vi "LatManClicks.vi"(9 "nMilliseconds":i32=2000, 10 "error in (no error)":errorcluster, 11 "On/OFF":bool) -> (2 "error out":errorcluster)   [LabVIEW 2014]
panel:
  in  "AutoItX3Lib.IAutoItX3":refnum<k7>
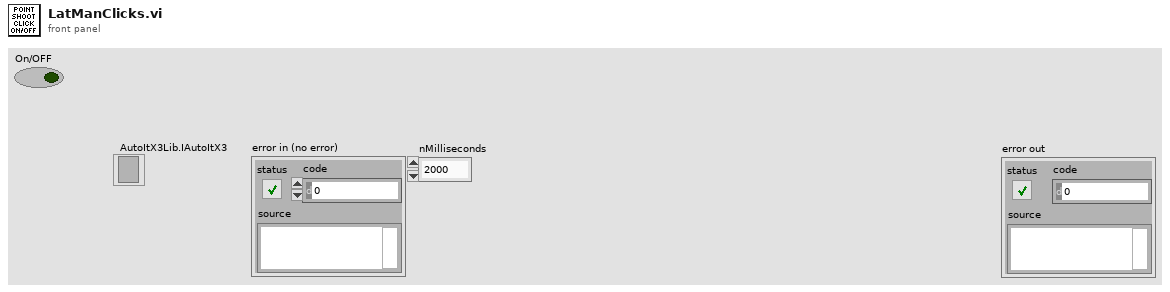
[diagram p1: front panel]
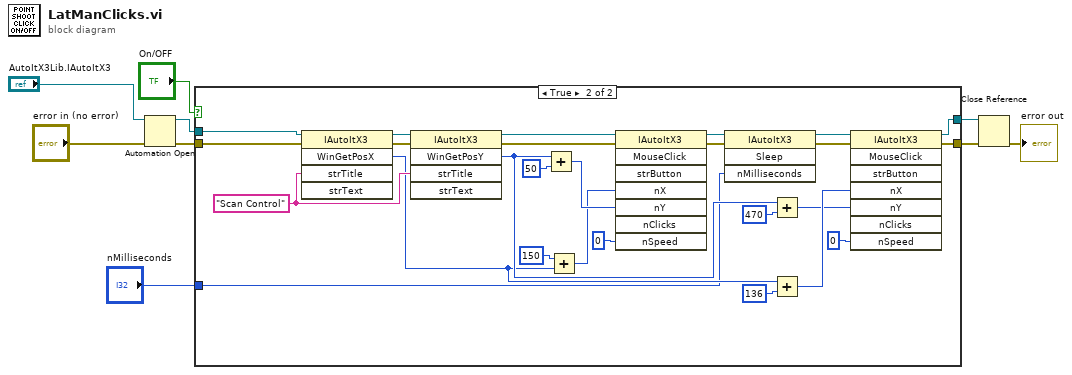
[diagram p0: block diagram]
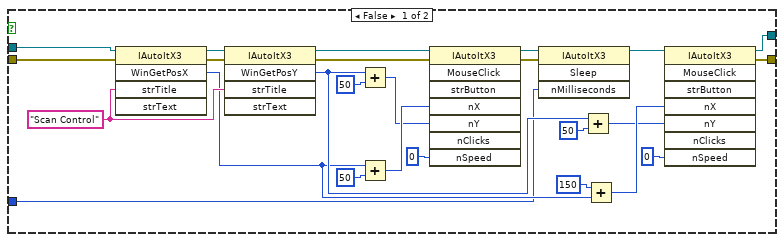
[diagram p2: hidden frame]
diagram:
  n1 = Automation Open(error in (no error)="error in (no error)", Automation Refnum="AutoItX3Lib.IAutoItX3") -> (Automation Refnum=w7:refnum<k7>, error out=w6:errorcluster)  [unwired: 2 in]
  n2 = case shown="True" "On/OFF" {
    tunnel: w7 -> [w32 w60]
    tunnel: w6 -> [w31 w59]
    tunnel: [w25 w50] -> w5
    tunnel: [w13 w49] -> w4
    tunnel: "nMilliseconds" -> [w10 w35]
    frame False {
      w24 = "Scan Control" ("strTitle")
      n3 = invoke class="IAutoItX3" method="WinGetPosX"(reference=w32, error in=w31, "strTitle"=w24) -> (reference out=w30:refnum<k7>, error out=w27:errorcluster, "WinGetPosX"=w22:i32)  [unwired: 2 in, 2 out]
      n4 = invoke class="IAutoItX3" method="WinGetPosY"(reference=w30, error in=w27, "strTitle"=w24) -> (reference out=w29:refnum<k7>, error out=w28:errorcluster, "WinGetPosY"=w23:i32)  [unwired: 2 in, 2 out]
      n5 = Add(x=w23, y=50) -> (x+y=w18:i32)
      n6 = Add(x=w22, y=50) -> (x+y=w19:i32)
      n7 = invoke class="IAutoItX3" method="MouseClick"(reference=w29, error in=w28, "nX"=w19, "nY"=w18, "nSpeed"=0) -> (reference out=w34:refnum<k7>, error out=w33:errorcluster)  [unwired: 3 in, 6 out]
      n8 = invoke class="IAutoItX3" method="Sleep"(reference=w34, error in=w33, "nMilliseconds"=w10) -> (reference out=w26:refnum<k7>)  [unwired: 1 in, 3 out]
      n9 = Add(x=w23, y=50) -> (x+y=w20:i32)
      n10 = Add(x=150, y=w22) -> (x+y=w21:i32)
      n11 = invoke class="IAutoItX3" method="MouseClick"(reference=w26, "nX"=w21, "nY"=w20, "nSpeed"=0) -> (reference out=w25:refnum<k7>, error out=w13:errorcluster)  [unwired: 4 in, 6 out]
    }
    frame True {
      w56 = "Scan Control" ("strTitle")
      n12 = invoke class="IAutoItX3" method="WinGetPosX"(reference=w60, error in=w59, "strTitle"=w56) -> (reference out=w58:refnum<k7>, error out=w57:errorcluster, "WinGetPosX"=w43:i32)  [unwired: 2 in, 2 out]
      n13 = invoke class="IAutoItX3" method="WinGetPosY"(reference=w58, error in=w57, "strTitle"=w56) -> (reference out=w41:refnum<k7>, error out=w40:errorcluster, "WinGetPosY"=w45:i32)  [unwired: 2 in, 2 out]
      n14 = Add(x=w45, y=50) -> (x+y=w48:i32)
      n15 = Add(x=150, y=w43) -> (x+y=w42:i32)
      n16 = invoke class="IAutoItX3" method="MouseClick"(reference=w41, error in=w40, "nX"=w42, "nY"=w48, "nSpeed"=0) -> (reference out=w39:refnum<k7>, error out=w38:errorcluster)  [unwired: 3 in, 6 out]
      n17 = invoke class="IAutoItX3" method="Sleep"(reference=w39, error in=w38, "nMilliseconds"=w35) -> (reference out=w37:refnum<k7>, error out=w36:errorcluster)  [unwired: 1 in, 2 out]
      n18 = Add(x=w45, y=470) -> (x+y=w54:i32)
      n19 = Add(x=w43, y=136) -> (x+y=w55:i32)
      n20 = invoke class="IAutoItX3" method="MouseClick"(reference=w37, error in=w36, "nX"=w55, "nY"=w54, "nSpeed"=0) -> (reference out=w50:refnum<k7>, error out=w49:errorcluster)  [unwired: 3 in, 6 out]
    }
  }
  n21 = Close Reference(reference=w5, error in (no error)=w4) -> (error out=→"error out":errorcluster)
